vi "Get Client Handler MTQ.vi"(8 "error in (no error)":errorcluster, 10 "GUID":string, 11 "Websocket Server in":refnum<class "Websocket Server.lvclass">) -> (0 "error out":errorcluster, 1 "Found?":bool, 2 "Websocket Client Handler MTQ":refnum<class "Message Transport Queue.lvclass">, 3 "Websocket Server out":refnum<class "Websocket Server.lvclass">)   [LabVIEW 2016, in "Stream Mediator.lvlib" / "Websocket Server.lvclass"]
uses:
  <userlib>/Composed Systems/Stream/Mediator/Classes/Websocket Server Actor/Websocket Server/Websocket Server.lvclass
  <userlib>/Composed Systems/Stream/Mediator/Classes/Message Transport Queue/Message Transport Queue.lvclass
  <userlib>/Composed Systems/Stream/Mediator/Classes/Websocket Server Actor/Websocket Server/Websocket Server.lvclass/Websocket Server.ctl
  <userlib>/Composed Systems/Stream/Mediator/Classes/Subscriber Look Up Table/Subscriber Look Up Table.lvclass
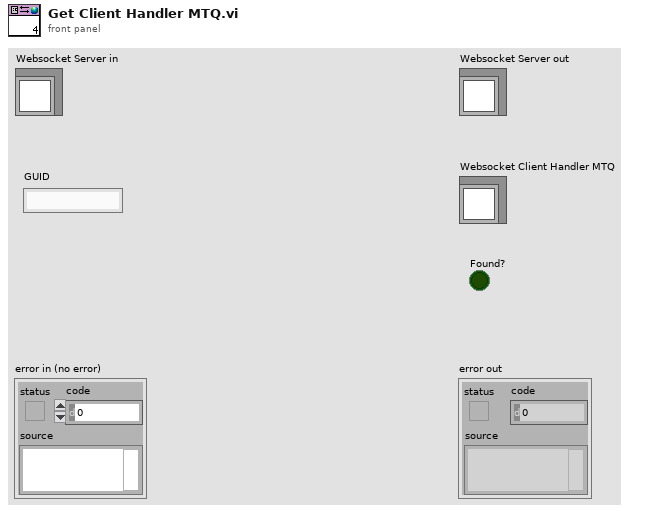
[diagram p1: front panel]
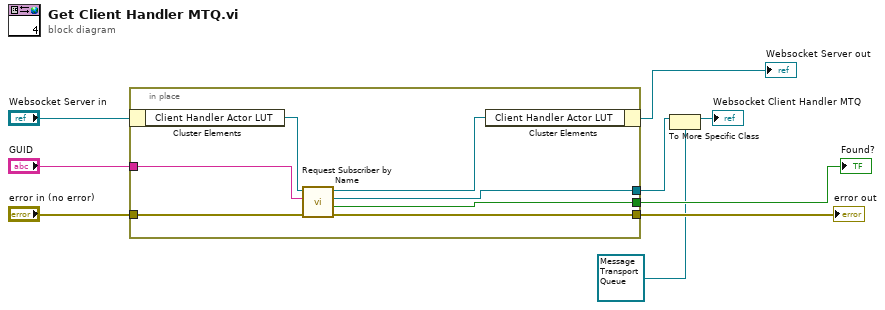
[diagram p0: block diagram]
diagram:
  n1 = in-place {
    in-place-border: "GUID" -> [w16]
    in-place-border: "error in (no error)" -> [w12]
    in-place-border: [w13] -> w5
    in-place-border: [w11] -> w3
    in-place-border: [w10] -> w4
    n2 = in-place-cluster #1("Websocket Server in") -> ("Client Handler Actor LUT"=w15:refnum<class "Subscriber Look Up Table.lvclass">)
    n3 = call <userlib>:"Request Subscriber by Name.vi"("error in (no error)"=w12, "Topic Name"=w16, "Subscriber Look Up Table in"=w15) -> ("error out"=w13:errorcluster, "Found?"=w10:bool, "Subscriber"=w11:refnum<class "Message Transport Interface.lvclass">, "Subscriber Look Up Table out"=w14:refnum<class "Subscriber Look Up Table.lvclass">)  [unwired: 5 in]
    n4 = in-place-cluster #1("Client Handler Actor LUT"=w14) -> (→"Websocket Server out":refnum<class "Websocket Server.lvclass">)
  }
  "error out" <- w5
  "Found?" <- w4
  n5 = To More Specific Class(target class=refnum<class "Message Transport Queue.lvclass"> refnum ("Stream Mediator.lvlib:Message Transport Queue.lvclass"), reference=w3) -> (specific class reference=→"Websocket Client Handler MTQ":refnum<class "Message Transport Queue.lvclass">)  [unwired: 1 in, 1 out]
